vi "Connect Channel.vi"(6 "Custom Channel Config Data":u8[](array[numeric]) format="%.0x", 8 "error in (no error)":errorcluster, 9 "Publisher Name":string, 10 "Subscriber Name":string, 11 "CIFChannelMng in":refnum<class "CIFChannelMng.lvclass">) -> (0 "error out":errorcluster, 3 "CIFChannelMng out":refnum<class "CIFChannelMng.lvclass">)   [LabVIEW 2021, in "CIFChannelMng.lvclass"]
uses:
  CIFChannelMng.lvclass
  CIFChannelMng.lvclass/CIFChannelMng.ctl
  CIFChannels/CIFChannels.lvclass/CIFChannels.ctl
  CIFChannels/Typedef/Channel State.ctl
  CIFChannels/Accessors/Read Channel State.vi
  ChannelCommon/Utilities/Add Error.vi
  <vilib>/CIF Foundation/CIF Utilities/Errors/Append Error Location.vi
  CIFChannels/CIFChannels.lvclass
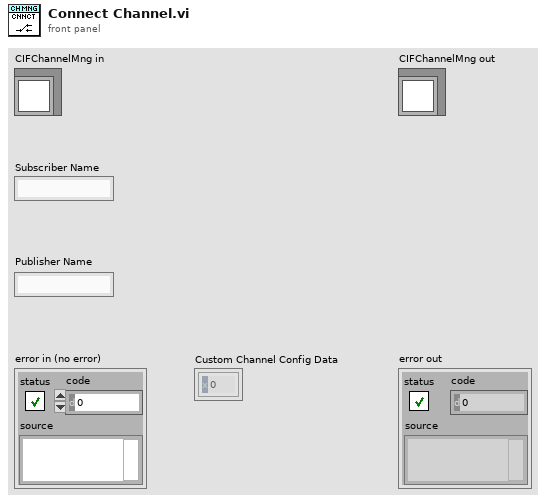
[diagram p1: front panel]
types:
  T1 = typedef "CIFChannels.lvclass/Channel State.ctl" = enum16{"Creating", "Disconnected", "Connecting", "Connected", "Destroyed"}
  T2 = typedef "CIFChannelMng.lvclass/Channel List for OOB.ctl" = cluster{"Name":string, "Direction":T3, "Type":string, "Connected?":bool, "Connected Name":string, "Custom Config Data":u8[], "Forced?":bool}
  T3 = typedef "CIFChannels.lvclass/Direction.ctl" = enum16{"Publisher", "Subscriber"}
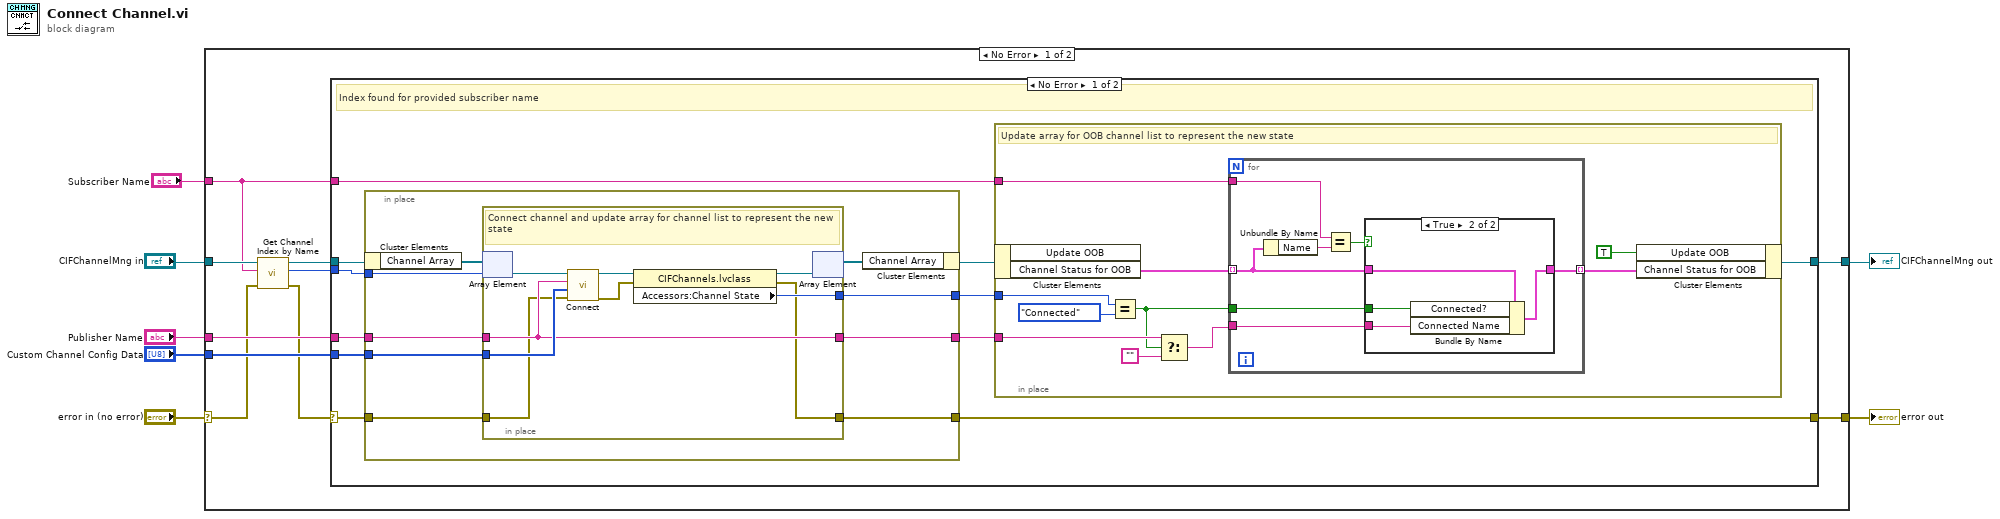
[diagram p0: block diagram]
diagram:
  n1 = case shown="No Error" "error in (no error)" {
    selector: "error in (no error)" -> [w14 w71]
    tunnel: [w9 w72] -> w5
    tunnel: "CIFChannelMng in" -> [w15 w72]
    tunnel: "Subscriber Name" -> [w10 _]
    tunnel: "Publisher Name" -> [w17 _]
    tunnel: "Custom Channel Config Data" -> [w16 _]
    tunnel: [w8 w71] -> w1
    frame No Error {
      n2 = call "Get Channel Index by Name.vi"("error in (no error)"=w14, "Channel Name"=w10, "CIFChannelMng in"=w15) -> ("error out"=w11:errorcluster, "Channel Index"=w12:i32, "CIFChannelMng out"=w13:refnum<class "CIFChannelMng.lvclass">)  [unwired: 6 in]
      n3 = case shown="No Error" w11 {
        selector: w11 -> [w24 w70]
        tunnel: w17 -> [w28 _]
        tunnel: w16 -> [w27 _]
        tunnel: w13 -> [w26 w69]
        tunnel: w12 -> [w25 _]
        tunnel: w10 -> [w20 _]
        tunnel: [w19 w69] -> w9
        tunnel: [w18 w70] -> w8
        frame No Error {
          # "Index found for provided subscriber name"
          n4 = in-place {
            in-place-border: w28 -> [w59]
            in-place-border: w27 -> [w58]
            in-place-border: [w56] -> w21
            in-place-border: [w57] -> w22
            in-place-border: w25 -> [w54]
            in-place-border: w24 -> [w53]
            in-place-border: [w51] -> w18
            n5 = in-place-cluster #1(w26) -> ("Channel Array"=w55:refnum<class "CIFChannels.lvclass">[])
            n6 = in-place {
              in-place-border: w59 -> [w64]
              in-place-border: w58 -> [w68]
              in-place-border: [w65] -> w57
              in-place-border: [w64] -> w56
              in-place-border: w53 -> [w62]
              in-place-border: [w60] -> w51
              # "Connect channel and update array for channel list to represent the new state"
              n7 = in-place-array #2(w55, w54) -> (w63:refnum<class "CIFChannels.lvclass">)
              n8 = call-dynamic "Connect.vi"("error in (no error)"=w62, "Custom Config Data"=w68, "Connection Name"=w64, "CIFChannels in"=w63) -> ("error out"=w66:errorcluster, "CIFChannels out"=w67:refnum<class "CIFChannels.lvclass">)  [unwired: 6 in]
              n9 = property class="CIFChannels.lvclass"(reference=w67, error in=w66) -> (reference out=w61:refnum<class "CIFChannels.lvclass">, error out=w60:errorcluster, "Accessors:Channel State"=w65:T1)
              n10 = in-place-array #2(w61) -> (w52:refnum<class "CIFChannels.lvclass">[])  [unwired: 1 out]
            }
            n11 = in-place-cluster #1("Channel Array"=w52) -> (w23:refnum<class "CIFChannelMng.lvclass">)
          }
          n12 = in-place {
            in-place-border: w21 -> [w37]
            in-place-border: w22 -> [w33]
            in-place-border: w20 -> [w29]
            # "Update array for OOB channel list to represent the new state"
            n13 = in-place-cluster #3(w23) -> ("Channel Status for OOB"=w32:T2[])  [unwired: 1 out]
            n14 = Equal?(x=w33, y=Channel_State."Connected") -> (x = y?=w35:bool)
            n15 = Select(t=w37, s=w35, f="") -> (s? t:f=w34:string)
            n16 = for {
              tunnel: w32 -> [w44] mode=indexing
              tunnel: w35 -> [w43]
              tunnel: w34 -> [w42]
              tunnel: [w41] -> w31 mode=indexing
              tunnel: w29 -> [w39]
              n17 = Unbundle By Name(w44) -> ("Name"=w45:string)
              n18 = Equal?(x=w39, y=w45) -> (x = y?=w40:bool)
              n19 = case shown="True" w40 {
                tunnel: w44 -> [w46 w50]
                tunnel: w43 -> [_ w49]
                tunnel: w42 -> [_ w48]
                tunnel: [w46 w47] -> w41
                frame False {
                }
                frame True {
                  n20 = Bundle By Name(cluster=w50, "Connected?"=w49, "Connected Name"=w48) -> (w47:T2)
                }
              }
            }
            n21 = in-place-cluster #3("Update OOB"=TRUE, "Channel Status for OOB"=w31) -> (w19:refnum<class "CIFChannelMng.lvclass">)
          }
        }
        frame Error {
          # "Index by name created error"
        }
      }
    }
    frame Error {
    }
  }
  "error out" <- w1
  "CIFChannelMng out" <- w5
